vi "Run.vi"(7 "Team Index":i32, 8 "Column":i32, 9 "Row":i32, 10 "View":i32[](array[numeric]) caption="View (Team Index, -1: empty)", 11 "DaveT In":refnum<class "DaveT.lvclass">) -> (0 "Replicated":refnum<class "Square.lvclass">, 1 "Direction":T1, 2 "Action":T2, 3 "Square Out":refnum<class "Square.lvclass">)   [LabVIEW 2015, in "DaveT.lvclass"]
uses:
  DaveT.lvclass
  Square/Square.lvclass
  Type Defs/Action Enum.ctl
  Type Defs/Direction Enum.ctl
  DaveT.lvclass/DaveT.ctl
  DaveT Purpose.ctl
  Type Defs/SB Type Defs.lvlib
panel:
  # "NW\nN\nNE\nE\nSE\nS\nSW\nW"
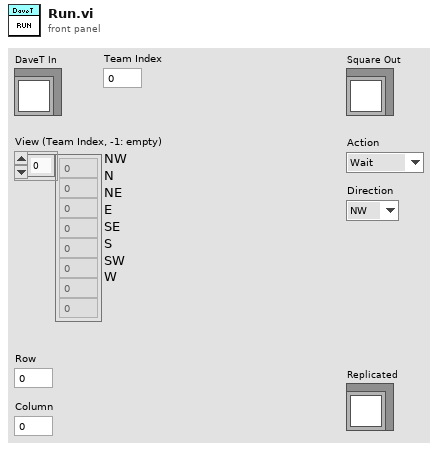
[diagram p1: front panel]
types:
  T1 = typedef "SB Type Defs.lvlib/Direction Enum.ctl" = enum16{"NW", "N", "NE", "E", "SE", "S", "SW", "W"}
  T2 = typedef "SB Type Defs.lvlib/Action Enum.ctl" = enum16{"Wait", "Move", "Attack", "Replicate"}
  T3 = typedef "DaveT.lvclass/DaveT Purpose.ctl" = enum16{"Spawn", "Attack", "Move"}
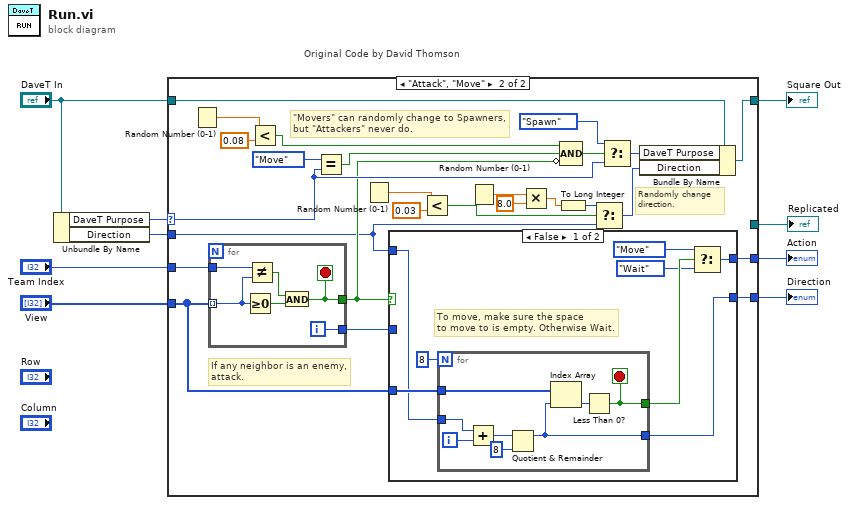
[diagram p0: block diagram]
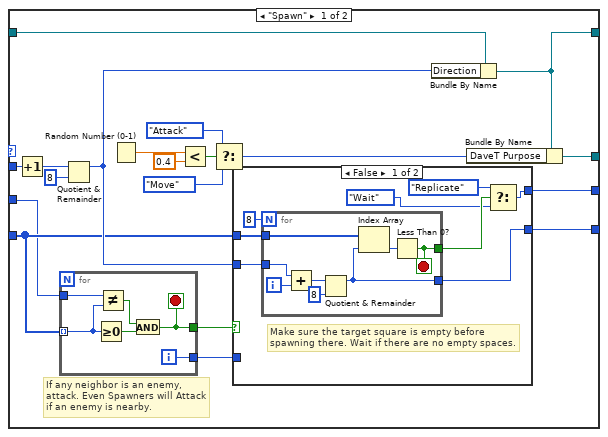
[diagram p2: hidden frame]
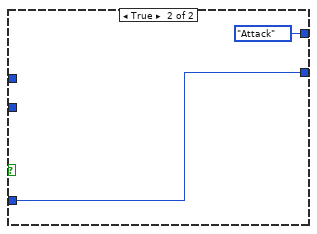
[diagram p3: hidden frame]
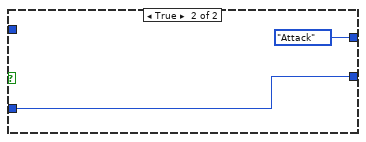
[diagram p4: hidden frame]
diagram:
  n1 = Unbundle By Name("DaveT In") -> ("DaveT Purpose"=w9:T3, "Direction"=w3:i32)
  n2 = case "Original Code by David Thomson" shown="\"Attack\", \"Move\"" w9 {
    selector: w9 -> [_ w66]
    tunnel: "DaveT In" -> [w24 w74]
    tunnel: [w23 w73] -> w7
    tunnel: [w28 w78] -> w6
    tunnel: [w11 w77] -> w5
    tunnel: [w22 _] -> w4
    tunnel: w3 -> [w27 w59]
    tunnel: "Team Index" -> [w13 w63]
    tunnel: "View" -> [w14 w62]
    frame "Spawn" {
      # "If any neighbor is an enemy,\nattack. Even Spawners will Attack\nif an enemy is nearby."
      n3 = Increment(x=w27) -> (x+1=w26:i32)
      n4 = for {
        tunnel: w14 -> [w50] mode=indexing
        tunnel: w13 -> [w49]
        tunnel: [w47] -> w12
        tunnel: [w48] -> w10
        i -> [w48]
        stop <- w47 stop-if-true
        n5 = Greater Or Equal To 0?(x=w50) -> (x >= 0?=w52:bool)
        n6 = Not Equal?(x=w49, y=w50) -> (x != y?=w51:bool)
        n7 = And(x=w51, y=w52) -> (x .and. y?=w47:bool)
      }
      n8 = Quotient & Remainder(x=w26, y=8) -> (x-y*floor(x/y)=w15:i32)  [unwired: 1 out]
      n9 = Random Number (0-1)() -> (number: 0 to 1=w21:dbl)
      n10 = Less?(x=w21, y=0.4) -> (x < y?=w17:bool)
      n11 = Select(t=DaveT_Purpose."Attack" ("DaveT Purpose"), s=w17, f=DaveT_Purpose."Move" ("DaveT Purpose")) -> (s? t:f=w16:T3)
      n12 = case shown="False" w12 {
        tunnel: [w31 Action_Enum."Attack" ("Action")] -> w28
        tunnel: w15 -> [w35 _]
        tunnel: w14 -> [w34 _]
        tunnel: [w30 w45] -> w11
        tunnel: w10 -> [_ w45]
        frame False {
          # "Make sure the target square is empty before\nspawning there. Wait if there are no empty spaces."
          n13 = for {
            N: 8 -> [_]
            tunnel: w34 -> [w41]
            tunnel: [w39] -> w32
            tunnel: [w38] -> w30
            tunnel: w35 -> [w37]
            i -> [w44]
            stop <- w39 stop-if-true
            n14 = Add(x=w37, y=w44) -> (x+y=w42:i32)
            n15 = Quotient & Remainder(x=w42, y=8) -> (x-y*floor(x/y)=w38:i32)  [unwired: 1 out]
            n16 = Index Array(array=w41, index=w38) -> (element=w40:i32)
            n17 = Less Than 0?(x=w40) -> (x < 0?=w39:bool)
          }
          n18 = Select(t=Action_Enum."Replicate" ("Action"), s=w32, f=Action_Enum."Wait" ("Action")) -> (s? t:f=w31:T2)
        }
        frame True {
        }
      }
      n19 = Bundle By Name(cluster=w24, "Direction"=w15) -> (w23:refnum<class "DaveT.lvclass">)
      n20 = Bundle By Name(cluster=w23, "DaveT Purpose"=w16) -> (w22:refnum<class "DaveT.lvclass">)
    }
    frame "Attack", "Move" {
      # "Randomly change\ndirection."
      # "\"Movers\" can randomly change to Spawners,\nbut \"Attackers\" never do."
      # "If any neighbor is an enemy,\nattack."
      n21 = Random Number (0-1)() -> (number: 0 to 1=w76:dbl)
      n22 = for {
        tunnel: w62 -> [w100] mode=indexing
        tunnel: w63 -> [w99]
        tunnel: [w97] -> w64
        tunnel: [w98] -> w70
        i -> [w98]
        stop <- w97 stop-if-true
        n23 = Greater Or Equal To 0?(x=w100) -> (x >= 0?=w102:bool)
        n24 = Not Equal?(x=w99, y=w100) -> (x != y?=w101:bool)
        n25 = And(x=w101, y=w102) -> (x .and. y?=w97:bool)
      }
      n26 = Less?(x=w76, y=0.08) -> (x < y?=w68:bool)
      n27 = Equal?(x=DaveT_Purpose."Move", y=w66) -> (x = y?=w67:bool)
      n28 = Random Number (0-1)() -> (number: 0 to 1=w60:dbl)
      n29 = case shown="False" w64 {
        tunnel: [w82 Action_Enum."Attack" ("Action")] -> w78
        tunnel: [w85 w95] -> w77
        tunnel: w59 -> [w80 _]
        tunnel: w70 -> [_ w95]
        tunnel: w62 -> [w86 _]
        frame False {
          # "To move, make sure the space\nto move to is empty. Otherwise Wait."
          n30 = for {
            N: 8 -> [_]
            tunnel: w86 -> [w91]
            tunnel: [w89] -> w84
            tunnel: [w88] -> w85
            tunnel: w80 -> [w87]
            i -> [w94]
            stop <- w89 stop-if-true
            n31 = Add(x=w87, y=w94) -> (x+y=w92:i32)
            n32 = Quotient & Remainder(x=w92, y=8) -> (x-y*floor(x/y)=w88:i32)  [unwired: 1 out]
            n33 = Index Array(array=w91, index=w88) -> (element=w90:i32)
            n34 = Less Than 0?(x=w90) -> (x < 0?=w89:bool)
          }
          n35 = Select(t=Action_Enum."Move" ("Action"), s=w84, f=Action_Enum."Wait" ("Action")) -> (s? t:f=w82:T2)
        }
        frame True {
        }
      }
      n36 = Less?(x=w60, y=0.03) -> (x < y?=w57:bool)
      n37 = Random Number (0-1)() -> (number: 0 to 1=w56:dbl)
      n38 = Multiply(x=w56, y=8.0) -> (x*y=w54:dbl)
      n39 = To Long Integer(number=w54) -> (32bit integer=w53:i32)
      n40 = Compound Arithmetic op=AND(w68, w67, invert w64) -> (w69:bool)
      n41 = Select(t=w53, s=w57, f=w59) -> (s? t:f=w58:i32)
      n42 = Select(t=DaveT_Purpose."Spawn" ("DaveT Purpose"), s=w69, f=w66) -> (s? t:f=w72:T3)
      n43 = Bundle By Name(cluster=w74, "DaveT Purpose"=w72, "Direction"=w58) -> (w73:refnum<class "DaveT.lvclass">)
    }
  }
  "Square Out" <- w7
  "Action" <- w6
  "Direction" <- w5
  "Replicated" <- w4
